vi "S_WriteAttribute.vi"(0 "reference in":refnum<class "SubTemplate.lvclass">, 5 "error in (no error)":errorcluster) -> (14 "reference out":refnum<class "SubTemplate.lvclass">, 19 "error out":errorcluster)   [LabVIEW 2012, in "SubTemplate.lvclass"]
uses:
  <resource>/Framework/Providers/Open_GDS/ClassProviders/Provider_EndevoGOOP300/Templates/SubTemplate/SubTemplate.lvclass
  <resource>/Framework/Providers/Open_GDS/ClassProviders/Provider_EndevoGOOP300/Templates/BaseTemplate/protected/ObjectAttributes.ctl
  <resource>/Framework/Providers/Open_GDS/ClassProviders/Provider_EndevoGOOP300/Templates/BaseTemplate/BaseTemplate.lvclass
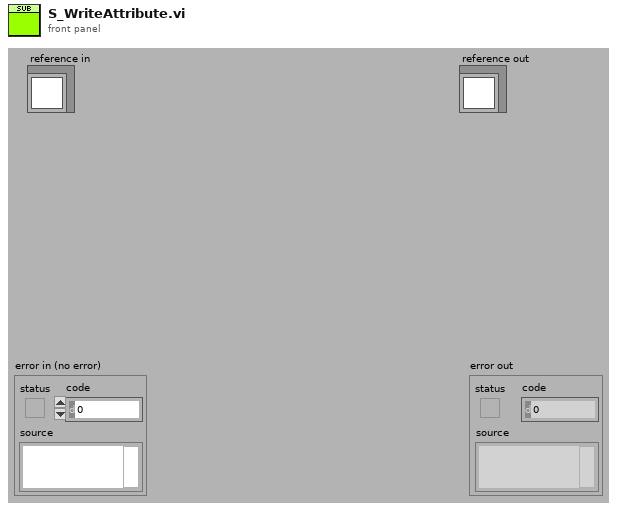
[diagram p1: front panel]
types:
  T1 = typedef "BaseTemplate.lvclass/ObjectAttributes.ctl" = cluster{"Attribute1":dbl}
  T2 = typedef "SubTemplate.lvclass/ObjectAttributes.ctl" = cluster{"Base class":T1}
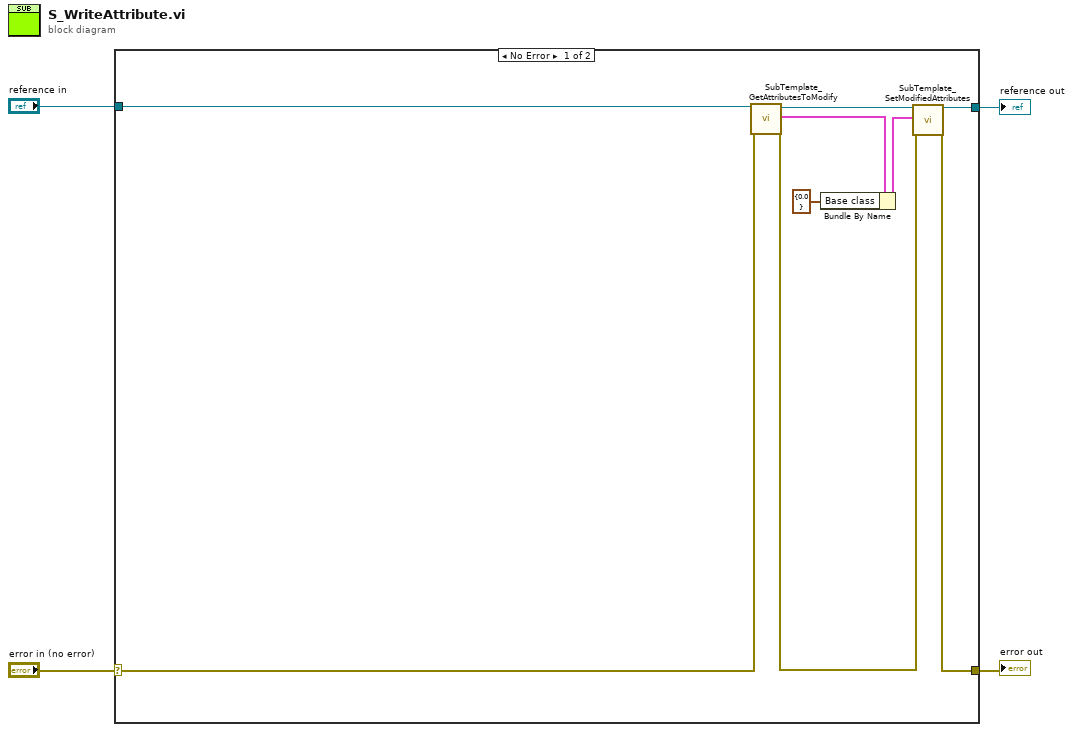
[diagram p0: block diagram]
diagram:
  n1 = case shown="No Error" "error in (no error)" {
    selector: "error in (no error)" -> [w8 w15]
    tunnel: [w10 w15] -> w3
    tunnel: [w7 w14] -> w1
    tunnel: "reference in" -> [w9 w14]
    frame No Error {
      n2 = call <resource>:"SubTemplate_GetAttributesToModify.vi"("reference in"=w9, "error in (no error)"=w8) -> ("reference out"=w11:refnum<class "SubTemplate.lvclass">, "Attributes"=w13:T2, "error out"=w6:errorcluster)  [unwired: 14 in, 1 out]
      n3 = Bundle By Name(cluster=w13, "Base class"=T1 {"Attribute1"=0.0}) -> (w12:T2)
      n4 = call <resource>:"SubTemplate_SetModifiedAttributes.vi"("reference in"=w11, "Attributes"=w12, "error in (no error)"=w6) -> ("reference out"=w7:refnum<class "SubTemplate.lvclass">, "error out"=w10:errorcluster)  [unwired: 15 in]
    }
    frame Error {
    }
  }
  "error out" <- w3
  "reference out" <- w1
